vi "Test Skip Test.vi"(8 "error in (no error)":errorcluster, 11 "LUnit Test Case V2 Test Double In":refnum<class "Test Case Test Double.lvclass">) -> (0 "error out":errorcluster, 3 "LUnit Test Case V2 Test Double Out":refnum<class "Test Case Test Double.lvclass">)   [LabVIEW 2020, in "Test Case Test Double.lvclass"]
uses:
  Test Case Test Double.lvclass
  C:/Git/astemes-lunit/source/Core/LUnit Test Case/LUnit Test Case V2.lvclass
  Core/LUnit Test Case/LUnit Test Case.lvclass/LUnit Test Case.ctl
  Test Case Test Double.lvclass/Test Case Test Double.ctl
  Core/LUnit Test Case/LUnit Test Case.lvclass
  C:/Git/astemes-lunit/source/Core/LUnit Test Case/LUnit Test Case.lvclass
  C:/Git/astemes-lunit/source/Core/Runnable/Runnable.lvclass
  C:/Git/astemes-lunit/source/Tests/Test Case Test Double/Test Case Test Double.lvclass
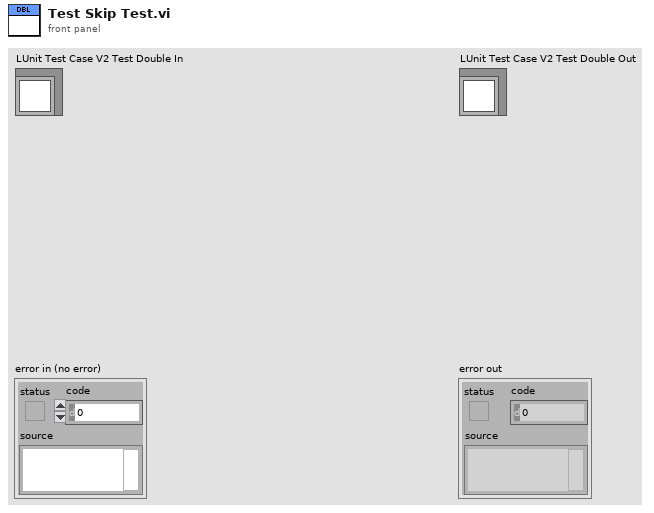
[diagram p1: front panel]
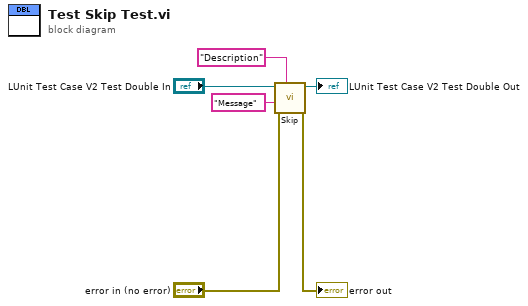
[diagram p0: block diagram]
diagram:
  n1 = call "Skip.vi"("Description"="Description", "error in (no error)"="error in (no error)", "Message"="Message", "LUnit Test Case In"="LUnit Test Case V2 Test Double In") -> ("error out"=→"error out":errorcluster, "LUnit Test Case Out"=→"LUnit Test Case V2 Test Double Out":refnum<class "Test Case Test Double.lvclass">)  [unwired: 6 in]
